vi "test.workspace_get.vi"   [LabVIEW 2020]
uses:
  Nominal Client/Nominal Client.lvclass/Nominal Client.ctl
  730c9c5b-7bb2-47cf-818b-6e2ed47344d4.vi
  Nominal Client/private_data.set.vi
  <vilib>/Utility/error.llb/Error Cluster From Error Code.vi
  submodules/reqwest-labview/lv-src/reqwest/create.vi
  Nominal Client/Palette Items/who_am_i.vi
  <vilib>/addons/_JKI Toolkits/Caraya/classes/Assert/Assert Greater Or Equal_Variant.vi
  <vilib>/addons/_JKI Toolkits/Caraya/classes/Assert/Assert Not Error.vi
  User/User.lvclass
  Nominal Client/Nominal Client.lvclass
  nominal types/workspace/workspace.lvclass
  submodules/reqwest-labview/lv-src/reqwest/reqwest.lvclass
  <vilib>/addons/_JKI Toolkits/Caraya/classes/Test/Test.lvclass
  <vilib>/addons/_JKI Toolkits/Caraya/classes/Assert/Assert.lvclass
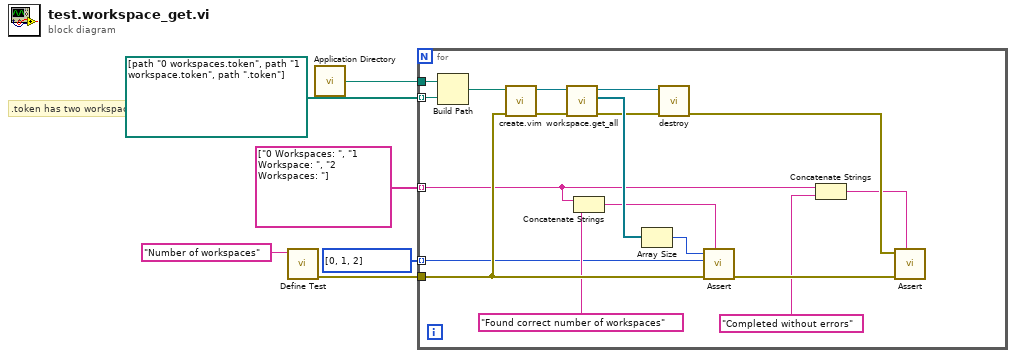
[diagram p0: block diagram]
diagram:
  # ".token has two workspaces"
  n1 = call <vilib>:"Define Test.vi"("Label (VI Title)"="Number of workspaces") -> ("error out"=w5:errorcluster)  [unwired: 9 in, 1 out]
  n2 = call <vilib>:"Application Directory.vi"() -> ("Application Directory"=w4:path)
  n3 = for {
    tunnel: w5 -> [w20]
    tunnel: w4 -> [w15]
    tunnel: path[] [path "0 workspaces.token", path "1 workspace.token", path ".token"] -> [w14] mode=indexing
    tunnel: string[] ["0 Workspaces: ", "1 Workspace: ", "2 Workspaces: "] ("Label") -> [w10] mode=indexing
    tunnel: i32[] [0, 1, 2] ("size(s)") -> [w7] mode=indexing
    n4 = Build Path(base path=w15, name or relative path=w14) -> (appended path=w13:path)
    n5 = call "create.vim"("error in"=w20, "API Token (string or path)"=w13) -> ("error out"=w23:errorcluster, "Nominal Client"=w24:refnum<class "Nominal Client.lvclass">)  [unwired: 7 in, 1 out]
    n6 = call "workspace.get_all.vi"("error in"=w23, "Nominal Client in"=w24) -> ("error out"=w19:errorcluster, "Workspaces"=w22:refnum<class "workspace.lvclass">[], "Nominal Client out"=w16:refnum<class "Nominal Client.lvclass">)  [unwired: 7 in]
    n7 = Concatenate Strings(w10, "Found correct number of workspaces" ("Label")) -> (w9:string)
    n8 = Array Size(array=w22) -> (size(s)=w21:i32)
    n9 = call "destroy.vi"("error in"=w19, "Nominal Client"=w16) -> ("error out"=w18:errorcluster)  [unwired: 9 in]
    n10 = call-poly <vilib>:"Assert.vi"("Label"=w9, "error in (no error)"=w20, "Y"=w7, "X"=w21) -> ("error out"=w17:errorcluster)  [unwired: 6 in, 1 out]
    n11 = Concatenate Strings(w10, "Completed without errors" ("Label")) -> (w8:string)
    n12 = call-poly <vilib>:"Assert.vi"("Label"=w8, "error in (no error)"=w17, "Not Error?"=w18) -> ()  [unwired: 7 in, 2 out]
  }
